vi "ArduinoPrimero.vi"() -> ()   [LabVIEW 2018]
uses:
  <vilib>/LabVIEW Interface for Arduino/Type Defs/Pin Mode.ctl
  <vilib>/LabVIEW Interface for Arduino/LabVIEW Interface for Arduino.lvlib
panel:
  in  "stop":bool
  in  "VISA Resource":string
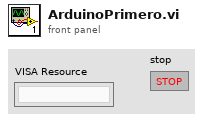
[diagram p1: front panel]
types:
  T1 = typedef "LabVIEW Interface for Arduino.lvlib/Arduino Resource.ctl" = cluster{"VISA resource":refnum<visa-resource-name>, "Board Type":T2, "Connection Type":enum8{"USB / Serial"}, "Bytes Per Packet (15)":u8}
  T2 = typedef "LabVIEW Interface for Arduino.lvlib/Board Type.ctl" = enum16{"Uno", "Dimuelanove w/Atmega 328", "Mega 2560"}
  T3 = typedef "LabVIEW Interface for Arduino.lvlib/Pin Mode.ctl" = enum8{"Input", "Output"}
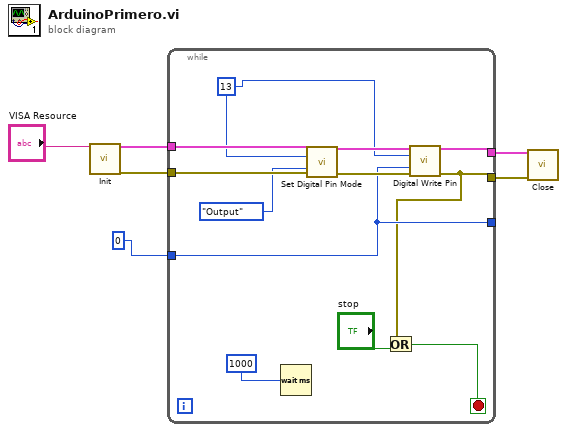
[diagram p0: block diagram]
diagram:
  n1 = call <vilib>:"Init.vi"("VISA resource"="VISA Resource") -> ("Arduino Resource"=w3:T1, "error out"=w4:errorcluster)  [unwired: 17 in]
  n2 = while {
    tunnel: [w15] -> w6
    tunnel: [w9] -> w5
    tunnel: w4 -> [w17]
    tunnel: w3 -> [w16]
    tunnel: 0 -> [w11]
    tunnel: [w11] -> _
    stop <- w10 stop-if-true
    w12 = 13
    n3 = Wait (ms)(milliseconds to wait=1000) -> ()  [unwired: 1 out]
    n4 = call <vilib>:"Set Digital Pin Mode.vi"("Arduino Resource"=w16, "Digital I/O Pin"=w12, "Pin Mode (Input)"=Pin_Mode."Output", "error in"=w17) -> ("Arduino Resource"=w13:T1, "error out"=w14:errorcluster)  [unwired: 10 in]
    n5 = call <vilib>:"Digital Write Pin.vi"("Arduino Resource"=w13, "Digital I/O Pin (0)"=w12, "Value (0)"=w11, "error in"=w14) -> ("Arduino Resource"=w15:T1, "error out"=w9:errorcluster)  [unwired: 10 in]
    n6 = Or(x=w9, y="stop") -> (x .or. y?=w10:bool)
  }
  n7 = call <vilib>:"Close.vi"("Arduino Resource"=w6, "error in"=w5) -> ()  [unwired: 13 in, 1 out]
